vi "Close emibin file.vi"(0 "refnum in":refnum<file>, 11 "error in (no error)":errorcluster) -> (15 "error out":errorcluster)   [LabVIEW 2011]
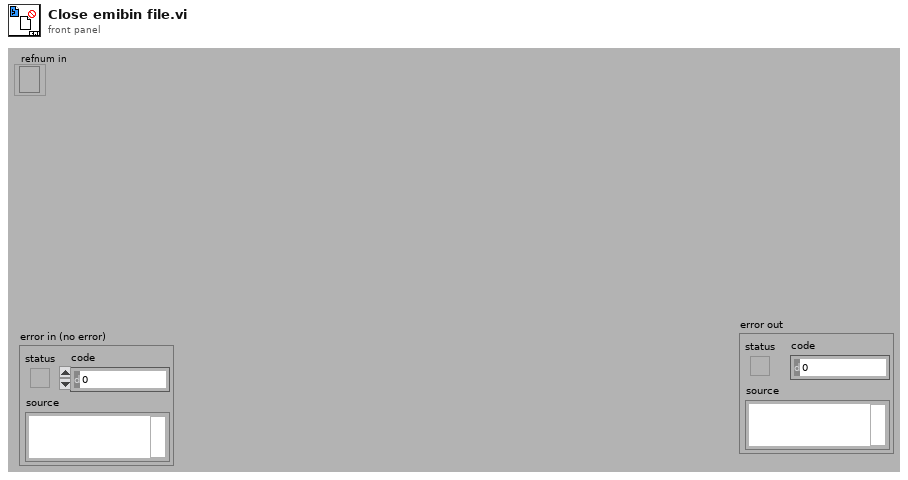
[diagram p1: front panel]
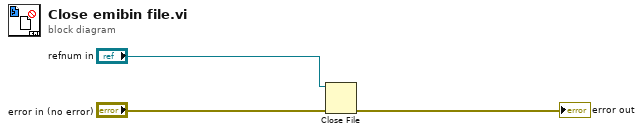
[diagram p0: block diagram]
diagram:
  n1 = Close File(refnum="refnum in", error in="error in (no error)") -> (error out=→"error out":errorcluster)  [unwired: 1 out]
